vi "Sequence.BuildMain.vi"(6 "Iterations":u32, 8 "error in (no error)":errorcluster, 9 "Sequence Channels":T1, 10 "Steps":T3[](array[typedef]), 11 "Sequence":refnum<k24>) -> (0 "error out":errorcluster, 3 "Sequence out":refnum<k24>)   [LabVIEW 2013, in "Simple Sequence Editor.lvlib"]
uses:
  Simple Sequence Editor.lvlib
  NationalInstruments.VeriStand.RealTimeSequenceDefinitionApi
  Types/Compiled.StepProperties.ctl
  Types/Compiled.IOStateProperties.ctl
  Types/Compiled.StepElementProperties.ctl
  Types/ChannelProperties.ctl
  Types/StepTypes.ctl
  Types/Compiled.StepCondition.ctl
  Types/OperationTypes.ctl
  Types/Compiled.SequenceChannels.ctl
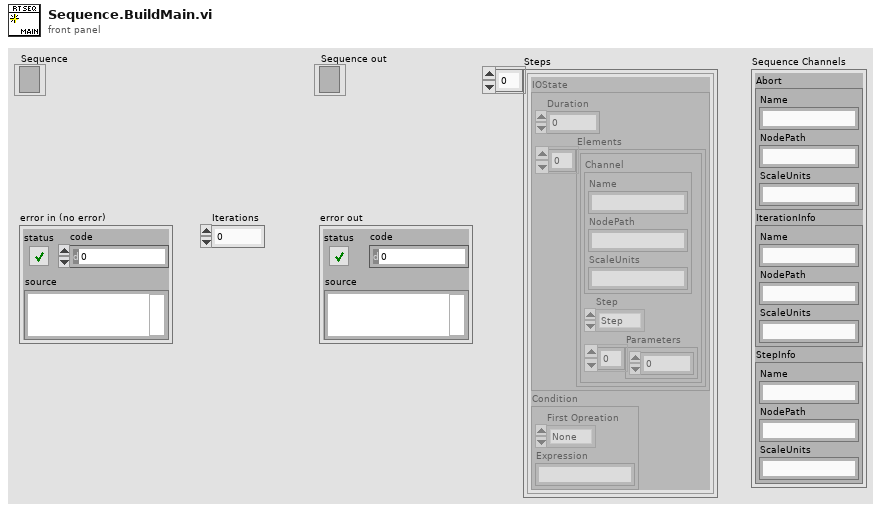
[diagram p1: front panel]
types:
  T1 = typedef "Simple Sequence Editor.lvlib/Compiled.SequenceChannels.ctl" = cluster{"Abort":T2, "IterationInfo":T2, "StepInfo":T2}
  T2 = typedef "Simple Sequence Editor.lvlib/ChannelProperties.ctl" = cluster{"Name":string, "NodePath":string, "ScaleUnits":string}
  T3 = typedef "Simple Sequence Editor.lvlib/Compiled.StepProperties.ctl" = cluster{"IOState":T4, "Condition":T7}
  T4 = typedef "Simple Sequence Editor.lvlib/Compiled.IOStateProperties.ctl" = cluster{"Duration":dbl, "Elements":T5[]}
  T5 = typedef "Simple Sequence Editor.lvlib/Compiled.StepElementProperties.ctl" = cluster{"Channel":T2, "Step":T6, "Parameters":dbl[]}
  T6 = typedef "Simple Sequence Editor.lvlib/StepTypes.ctl" = enum8{"Step", "iStep", "Ramp", "Unchanged", "Unknown"}
  T7 = typedef "Simple Sequence Editor.lvlib/Compiled.StepCondition.ctl" = cluster{"First Opreation":T8, "Expression":string}
  T8 = typedef "Simple Sequence Editor.lvlib/OperationTypes.ctl" = enum8{"None", "&&", "||"}
  T9 = typedef "Simple Sequence Editor.lvlib/Sequence.MainSeqRefs.ctl" = cluster{"Task.Main":refnum<k24>, "For.Main":refnum<k24>, "While.Main":refnum<k24>, "SelectCases.Main":refnum<k24>, "Select.Main":refnum<k24>}
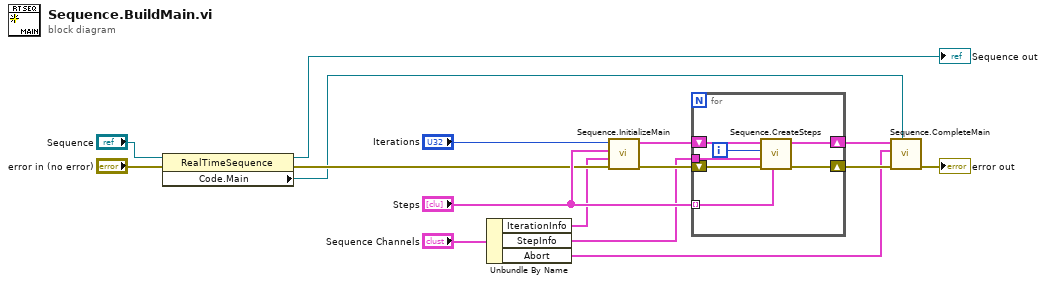
[diagram p0: block diagram]
diagram:
  n1 = property class="RealTimeSequence"(reference="Sequence", error in="error in (no error)") -> (reference out=→"Sequence out":refnum<k24>, error out=w9:errorcluster, "Code.Main"=w1:refnum<k24>)
  n2 = Unbundle By Name("Sequence Channels") -> ("IterationInfo"=w6:T2, "StepInfo"=w4:T2, "Abort"=w2:T2)
  n3 = call "Sequence.InitializeMain.vi"("error in (no error)"=w9, "IterationInfo"=w6, "Steps"="Steps", "Iterations"="Iterations") -> ("error out"=w13:errorcluster, "Refs"=w5:T9)  [unwired: 6 in]
  n4 = for {
    tunnel: "Steps" -> [w23] mode=indexing
    shift-right: [w22] -> w14
    shift-left: w13 -> [w19]
    tunnel: w4 -> [w20]
    shift-right: [w17] -> w3
    shift-left: w5 -> [w18]
    i -> [w21]
    n5 = call "Sequence.CreateSteps.vi"("Step"=w23, "error in (no error)"=w19, "StepInfo"=w20, "Numeric"=w21, "Refs"=w18) -> ("error out"=w22:errorcluster, "Refs out"=w17:T9)  [unwired: 5 in]
  }
  n6 = call "Sequence.CompleteMain.vi"("Code.Main"=w1, "error in (no error)"=w14, "Abort"=w2, "Refs"=w3) -> ("error out"=→"error out":errorcluster)  [unwired: 7 in]
